vi "ARRAY.vi"() -> ()   [LabVIEW 2017]
panel:
  out "x+y":dbl[][][](array[numeric])
  in  "INPUT 2":dbl[][][](array[numeric])
  in  "INPUT1":dbl[][][](array[numeric])
  # "1D ARRAY"
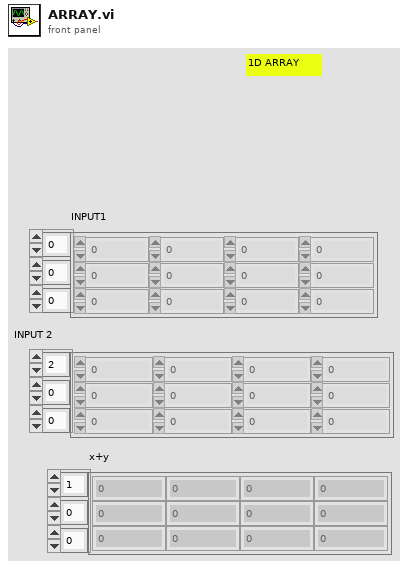
[diagram p1: front panel]
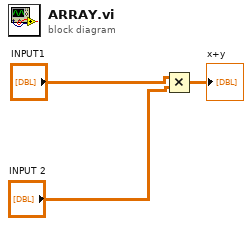
[diagram p0: block diagram]
diagram:
  n1 = Multiply(x="INPUT1", y="INPUT 2") -> (x*y=→"x+y":dbl[][][])
